vi "queue combined test.vi"() -> ()   [LabVIEW 2015]
uses:
  connection/connection maintainer.lvclass
  message/communicator message.lvclass
  communicator/communicator.lvclass/communicator.ctl
  Queue server/Queue server.lvclass
  Queue Client/Queue client.lvclass
  communicator/communicator.lvclass
panel:
  in  "data 4":string
  in  "ID 4":string
  in  "data 3":string
  in  "ID 3":string
  out "data 2":variant
  out "ID 2":string
  out "data":variant
  out "ID":string
  out "error out":errorcluster
  out "server":refnum<class "connection maintainer.lvclass">
  out "client":refnum<class "connection maintainer.lvclass">
  in  "remake s":bool
  in  "remake c":bool
  in  "S to C":bool
  in  "C to S":bool
  in  "exits":bool
  out "ClienT":timestamp
  out "servT":timestamp
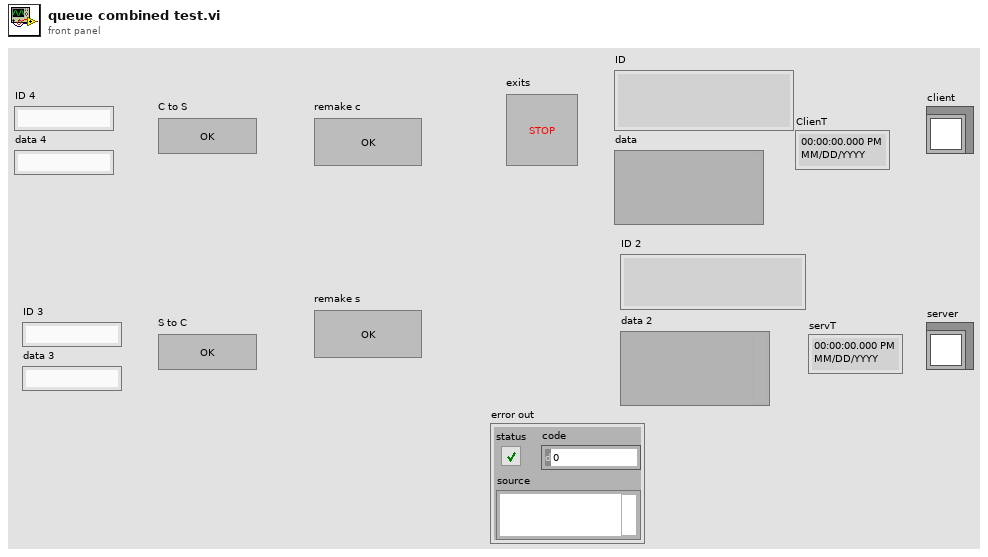
[diagram p1: front panel]
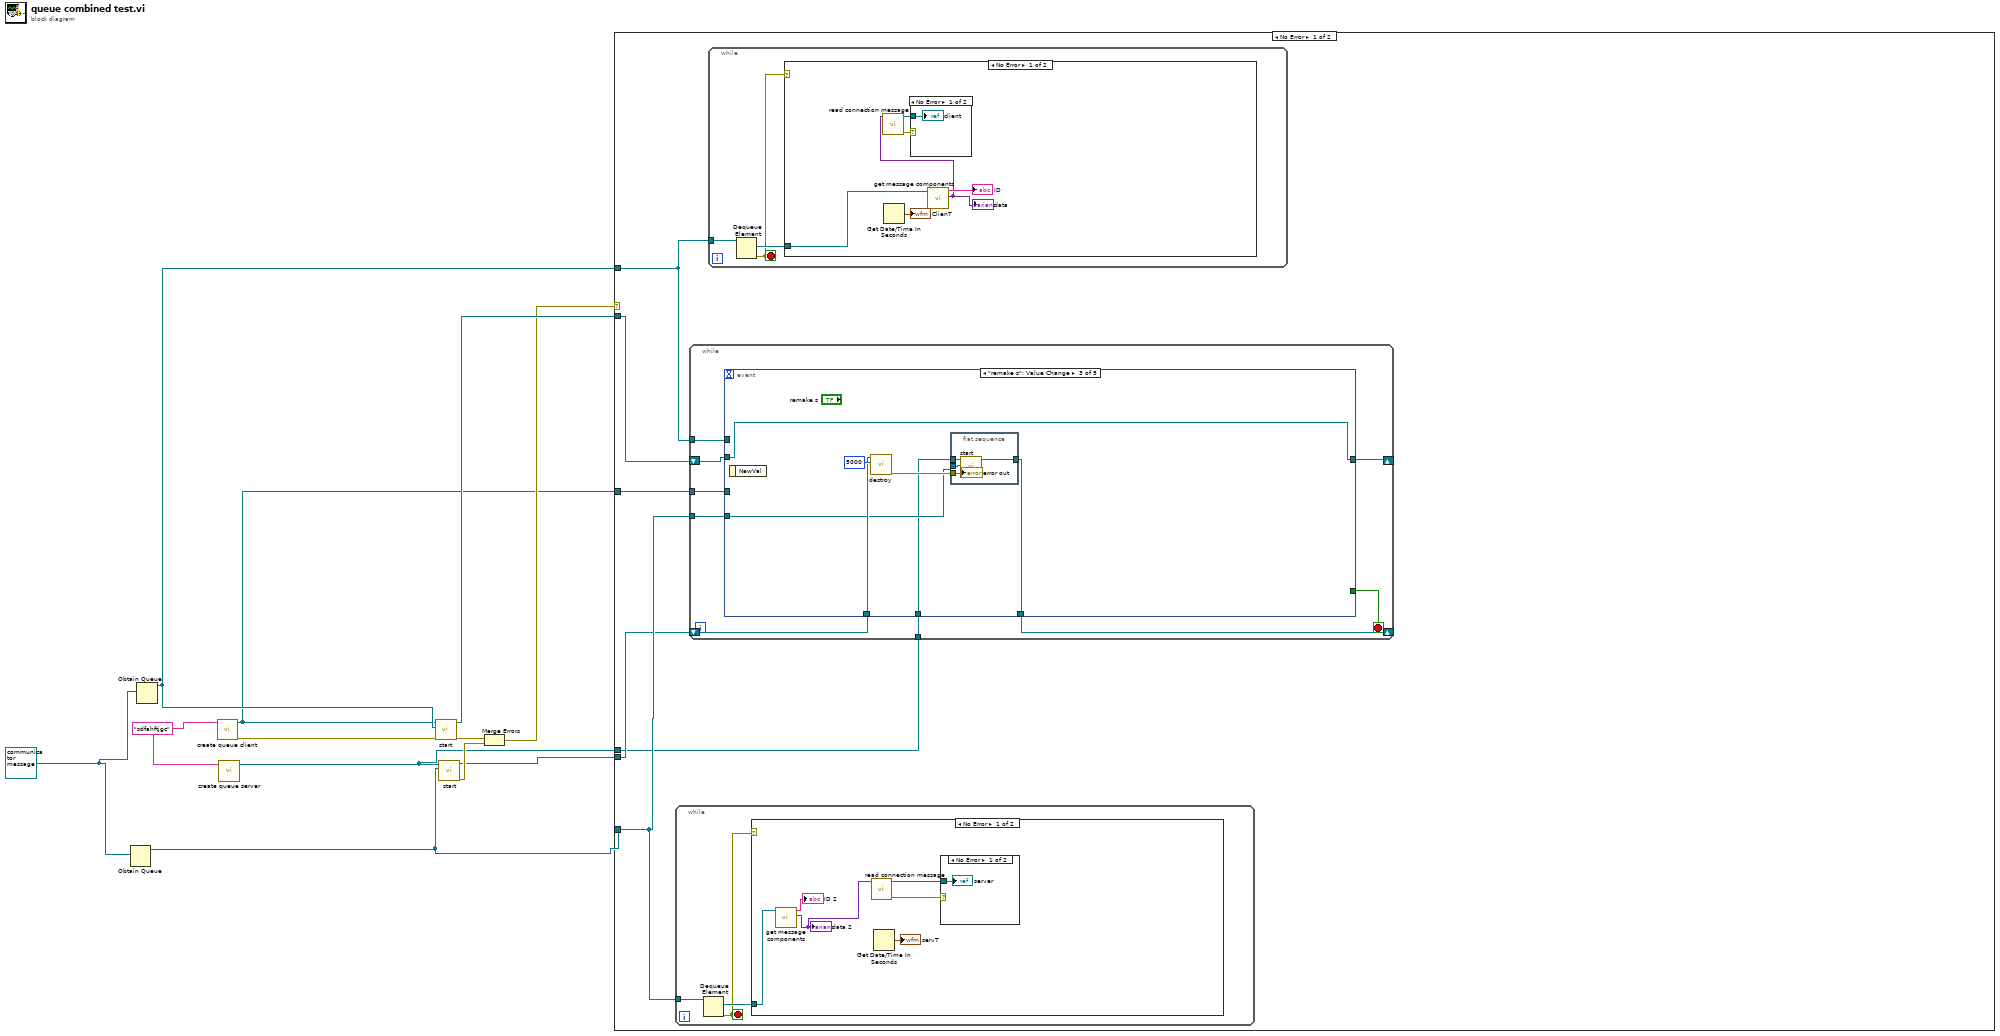
[diagram p0: block diagram]
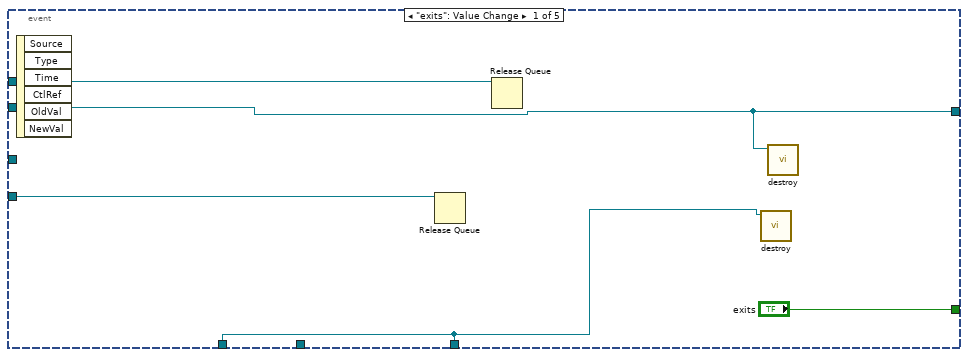
[diagram p2: hidden frame]
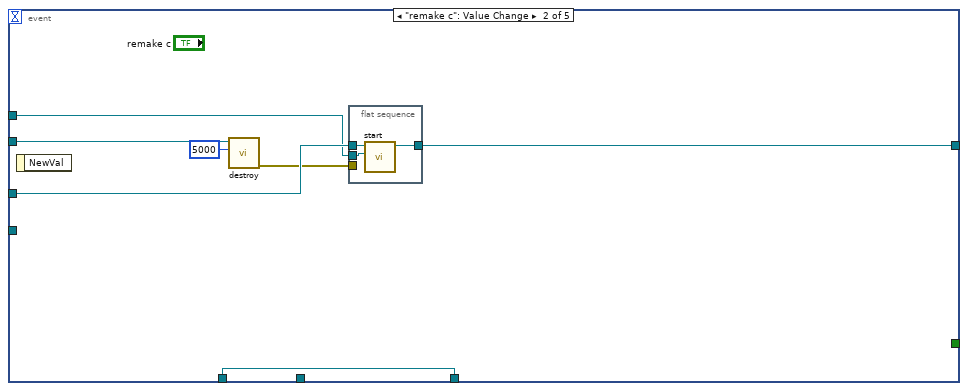
[diagram p3: hidden frame]
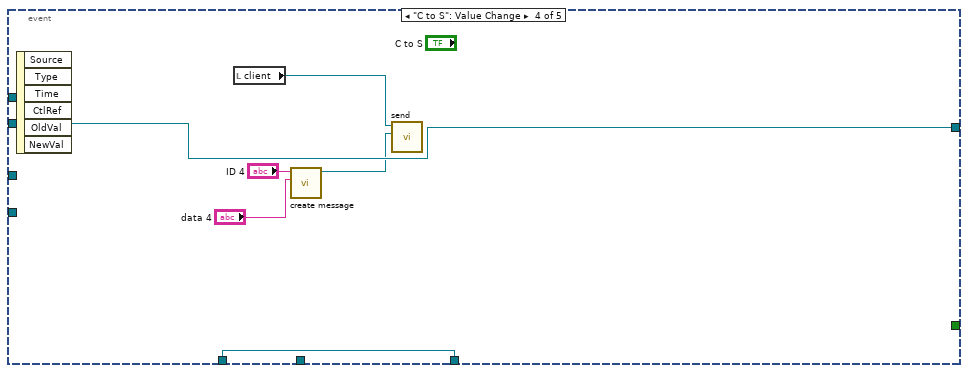
[diagram p4: hidden frame]
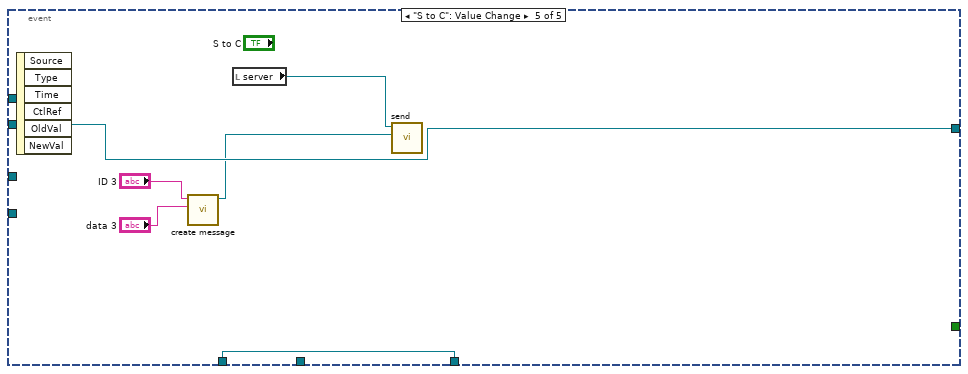
[diagram p5: hidden frame]
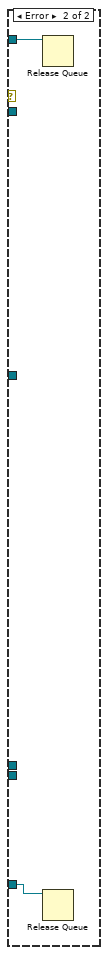
[diagram p10: hidden frame]
diagram:
  w1 = refnum<class "communicator message.lvclass"> refnum ("message")
  w9 = "sdfahftjgc" ("connection string")
  n1 = Obtain Queue(element data type=w1) -> (queue out=w5:refnum<queue>)  [unwired: 4 in, 2 out]
  n2 = Obtain Queue(element data type=w1) -> (queue out=w6:refnum<queue>)  [unwired: 4 in, 2 out]
  n3 = call "create queue client.vi"("conn string"=w9) -> ("error out"=w12:errorcluster, "TCP client out"=w3:refnum<class "Queue client.lvclass">)  [unwired: 9 in]
  n4 = call "create queue server.vi"("conn string"=w9) -> ("TCP server out"=w2:refnum<class "Queue server.lvclass">)  [unwired: 9 in, 1 out]
  n5 = call-dynamic "start.vi"("error in"=w12, "queue to parent"=w6, "communicator in"=w3) -> ("error out"=w10:errorcluster, "communicator out"=w11:refnum<class "Queue client.lvclass">)  [unwired: 7 in]
  n6 = call-dynamic "start.vi"("queue to parent"=w5, "communicator in"=w2) -> ("error out"=w7:errorcluster, "communicator out"=w4:refnum<class "Queue server.lvclass">)  [unwired: 8 in]
  n7 = Merge Errors(w10, w7) -> (w8:errorcluster)
  n8 = case shown="No Error" w8 {
    tunnel: w6 -> [w17 w87]
    tunnel: w11 -> [w16 _]
    tunnel: w5 -> [w18 w86]
    tunnel: w4 -> [w14 _]
    tunnel: w3 -> [w15 _]
    tunnel: w2 -> [w13 _]
    frame No Error {
      n9 = while {
        tunnel: w18 -> [w68]
        stop <- w66 stop-if-true
        n10 = Dequeue Element(queue=w68) -> (element=w67:refnum<class "communicator message.lvclass">, error out=w66:errorcluster)  [unwired: 2 in, 2 out]
        n11 = case shown="No Error" w66 {
          tunnel: w67 -> [w69 _]
          frame No Error {
            n12 = call "get message components.vi"("message"=w69) -> ("data"=w70:variant, "ID"=→"ID 2":string)  [unwired: 9 in]
            "data 2" <- w70
            n13 = call "read connection message.vi"("data"=w70) -> ("error out"=w73:errorcluster, "conn"=w72:refnum<class "connection maintainer.lvclass">)  [unwired: 9 in]
            n14 = Get Date/Time In Seconds() -> (seconds since 1Jan1904=→"servT":timestamp)
            n15 = case shown="No Error" w73 {
              tunnel: w72 -> [w75 _]
              frame No Error {
                "server" <- w75
              }
              frame Error {
              }
            }
          }
          frame Error {
          }
        }
      }
      n16 = while {
        tunnel: w18 -> [w26]
        tunnel: w17 -> [w25]
        tunnel: w15 -> [w23]
        tunnel: w13 -> [w21]
        shift-right: [w20] -> _
        shift-left: w14 -> [w22]
        shift-right: [w19] -> _
        shift-left: w16 -> [w24]
        stop <- w27 stop-if-true
        n17 = event shown="[2] \"remake s\": Value Change" {
          selector: _ -> [_ _ _ _ _]
          dyn-events: _ -> [_ _ _ _ _]
          timeout: _ -> [_ _ _ _ _]
          tunnel: ["exits" _ _ _ _] -> w27
          tunnel: w26 -> [w31 _ w46 _ _]
          tunnel: w25 -> [w30 w35 _ _ _]
          tunnel: w24 -> [w28 w39 w43 w58 w64]
          tunnel: w23 -> [_ w38 _ _ _]
          tunnel: w22 -> [w29 w34 w47 w59 w65]
          tunnel: w21 -> [_ _ w45 _ _]
          tunnel: [w29 w34 w44 w59 w65] -> w20
          tunnel: [w28 w33 w43 w58 w64] -> w19
          event "exits": Value Change {
            n18 = event-data() -> ()  [unwired: 1 in, 6 out]
            n19 = Release Queue(queue=w31) -> ()  [unwired: 2 in, 3 out]
            n20 = Release Queue(queue=w30) -> ()  [unwired: 2 in, 3 out]
            n21 = call-dynamic "destroy.vi"("communicator in"=w29) -> ()  [unwired: 10 in, 1 out]
            n22 = call-dynamic "destroy.vi"("communicator in"=w28) -> ()  [unwired: 10 in, 1 out]
          }
          event "remake c": Value Change {
            n23 = event-data() -> ()  [unwired: 1 in, 1 out]
            n24 = call-dynamic "destroy.vi"("timeout in ms (-1)"=5000, "communicator in"=w39) -> ("error out"=w37:errorcluster)  [unwired: 9 in]
            n25 = flat-sequence {
              tunnel: w38 -> [w42]
              tunnel: w37 -> [_]
              tunnel: w35 -> [w41]
              tunnel: [w40] -> w33
              frame #0 {
                n26 = call-dynamic "start.vi"("queue to parent"=w41, "communicator in"=w42) -> ("communicator out"=w40:refnum<class "Queue client.lvclass">)  [unwired: 8 in, 1 out]
              }
            }
          }
          event "remake s": Value Change {
            n27 = event-data() -> ()  [unwired: 1 in, 1 out]
            n28 = call-dynamic "destroy.vi"("timeout in ms (-1)"=5000, "communicator in"=w47) -> ("error out"=w49:errorcluster)  [unwired: 9 in]
            n29 = flat-sequence {
              tunnel: w45 -> [w53]
              tunnel: w49 -> [w50]
              tunnel: w46 -> [w52]
              tunnel: [w51] -> w44
              frame #0 {
                n30 = call-dynamic "start.vi"("queue to parent"=w52, "communicator in"=w53) -> ("communicator out"=w51:refnum<class "Queue server.lvclass">)  [unwired: 8 in, 1 out]
                "error out" <- w50
              }
            }
          }
          event "C to S": Value Change {
            n31 = event-data() -> ()  [unwired: 1 in, 6 out]
            n32 = local read "client"() -> (w57:refnum<class "connection maintainer.lvclass">)
            n33 = call "create message.vi"("data"="data 4", "ID"="ID 4") -> ("message"=w54:refnum<class "communicator message.lvclass">)  [unwired: 9 in]
            n34 = call "send.vi"("element"=w54, "communicator in"=w57) -> ()  [unwired: 9 in, 1 out]
          }
          event "S to C": Value Change {
            n35 = event-data() -> ()  [unwired: 1 in, 6 out]
            n36 = call "create message.vi"("data"="data 3", "ID"="ID 3") -> ("message"=w60:refnum<class "communicator message.lvclass">)  [unwired: 9 in]
            n37 = local read "server"() -> (w63:refnum<class "connection maintainer.lvclass">)
            n38 = call "send.vi"("element"=w60, "communicator in"=w63) -> ()  [unwired: 9 in, 1 out]
          }
        }
      }
      n39 = while {
        tunnel: w17 -> [w78]
        stop <- w76 stop-if-true
        n40 = Dequeue Element(queue=w78) -> (element=w77:refnum<class "communicator message.lvclass">, error out=w76:errorcluster)  [unwired: 2 in, 2 out]
        n41 = case shown="No Error" w76 {
          tunnel: w77 -> [w79 _]
          frame No Error {
            n42 = Get Date/Time In Seconds() -> (seconds since 1Jan1904=→"ClienT":timestamp)
            n43 = call "get message components.vi"("message"=w79) -> ("data"=w80:variant, "ID"=→"ID":string)  [unwired: 9 in]
            "data" <- w80
            n44 = call "read connection message.vi"("data"=w80) -> ("error out"=w82:errorcluster, "conn"=w83:refnum<class "connection maintainer.lvclass">)  [unwired: 9 in]
            n45 = case shown="No Error" w82 {
              tunnel: w83 -> [w85 _]
              frame No Error {
                "client" <- w85
              }
              frame Error {
              }
            }
          }
          frame Error {
          }
        }
      }
    }
    frame Error {
      n46 = Release Queue(queue=w87) -> ()  [unwired: 2 in, 3 out]
      n47 = Release Queue(queue=w86) -> ()  [unwired: 2 in, 3 out]
    }
  }
